vi "Busy Indicator.vi"() -> ()   [LabVIEW 2011]
doc: "Busy Indicator.vi\n\n<B>Description:</B>\n\nThis VI is shown while the calling VI is busy. This VI is a modified version of TestStand - Busy Indicator.vi.\n\n<B>Usage:</B>\n\nNone.\n\n<B>NOTES:</B>\n\nNone.\n\n<B>Inputs:</B>\n\nNone.\n\n<B>Outputs:</B>\n\nNone.\n\n<B>Initial Developer:</B>\n\nNational Instruments\n\n<B>Modified by:</B>\n\nMark Ridgley\nMark.Ridgley_LabVIEW.Developer@comcast.net"
panel:
  out "Busy":u16(ring)
  in  "stop":bool
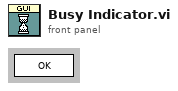
[diagram p1: front panel]
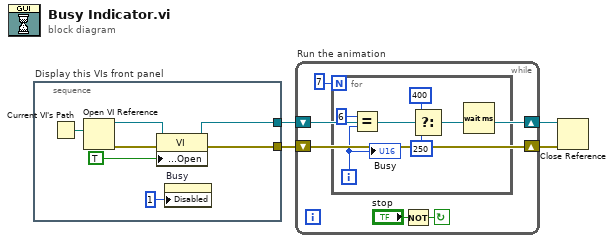
[diagram p0: block diagram]
diagram:
  n1 = stacked-sequence "Display this VIs front panel" {
    tunnel: [w11] -> w4
    tunnel: [w10] -> w3
    frame #0 {
      n2 = Current VI's Path() -> (path=w9:path)
      n3 = Open VI Reference(vi path=w9) -> (vi reference=w7:refnum<vi>, error out=w8:errorcluster)  [unwired: 5 in]
      n4 = property class="VI"(reference=w7, error in=w8, "Front Panel Window:Open"=TRUE ("Front Panel.Open")) -> (reference out=w11:refnum<vi>, error out=w10:errorcluster)
      n5 = property on="Busy" class="Ring (strict)"("Disabled"=u8 1) -> ()  [unwired: 2 in, 2 out]
    }
  }
  n6 = while "Run the animation" {
    shift-left: w4 -> [w12]
    shift-right: [w12] -> w1
    shift-left: w3 -> [w13]
    shift-right: [w13] -> w2
    stop <- w14 continue-if-true
    n7 = for {
      N: 7 -> [_]
      i -> [w18]
      n8 = Equal?(x=6, y=w18) -> (x = y?=w19:bool)
      n9 = Select(t=400, s=w19, f=250) -> (s? t:f=w20:i32)
      n10 = Wait (ms)(milliseconds to wait=w20) -> ()  [unwired: 1 out]
      "Busy" <- w18
    }
    n11 = Not(x="stop") -> (.not. x?=w14:bool)
  }
  n12 = Close Reference(reference=w1, error in (no error)=w2) -> ()  [unwired: 1 out]
